vi "3DS Light.vi"(8 "error in (no error)":errorcluster, 9 "Direction":cluster{"X":sgl, "Y":sgl, "Z":sgl}, 10 "Color":u32, 11 "SceneObject in":refnum<vi>) -> (0 "error out":errorcluster, 3 "SceneObject out":refnum<vi>)   [LabVIEW 2019, in "3D utilities.lvlib"]
uses:
  3D utilities.lvlib
  <vilib>/Utility/miscctls.llb/LV3DPointTypeDef.ctl
  <vilib>/picture/3D Picture Control/Helpers/Set Light (reference).vi
  <vilib>/picture/3D Picture Control/NI_3D Picture Control.lvlib
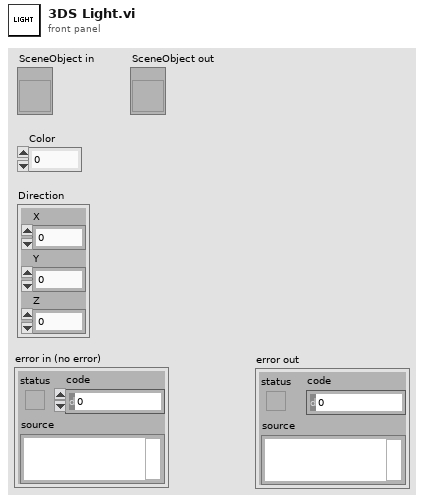
[diagram p1: front panel]
types:
  T1 = typedef "LV3DPointTypeDef.ctl" = cluster{"X":sgl, "Y":sgl, "Z":sgl}
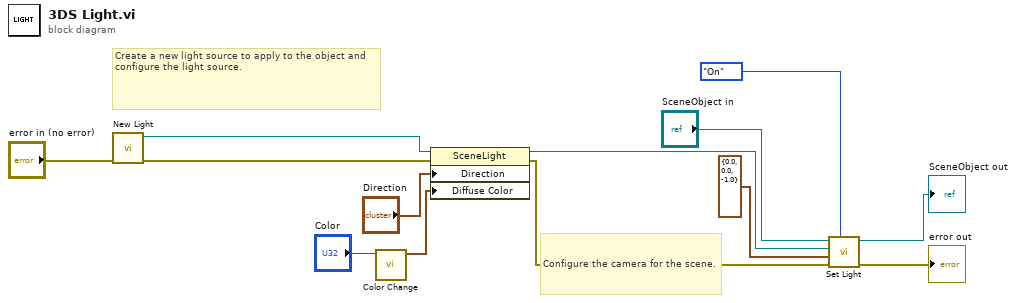
[diagram p0: block diagram]
diagram:
  # "Configure the camera for the scene."
  # "Create a new light source to apply to the object and configure the light source."
  n1 = call <vilib>:"New Light.vi"("error in (no error)"="error in (no error)") -> ("error out"=w8:errorcluster, "New Light Refnum"=w3:refnum<vi>)  [unwired: 2 in, 7 out]
  n2 = call <vilib>:"Color Change.vi"("Color"="Color") -> ("RGBA"=w10:cluster{"R":sgl, "G":sgl, "B":sgl, "A":sgl})  [unwired: 10 in]
  n3 = property class="SceneLight"(reference=w3, error in=w8, "Direction"="Direction", "Diffuse Color"=w10) -> (reference out=w6:refnum<vi>, error out=w13:errorcluster)
  n4 = call-poly <vilib>:"Set Light.vi"("Light State"=enum16{"Inherit Value", "Off", "On"}."On", "error in (no error)"=w13, "Position"=T1 {"X"=0.0, "Y"=0.0, "Z"=-1.0}, "Light Refnum In"=w6, "Scene Object In"="SceneObject in") -> ("error out"=→"error out":errorcluster, "Scene Object Out"=→"SceneObject out":refnum<vi>)  [unwired: 4 in, 1 out]
